vi "UTC KML time.vi"() -> (14 "String":string)   [LabVIEW 2015, in "Biblioteka moduł map v3.lvlib" / "KML.lvlib"]
uses:
  KML.lvlib
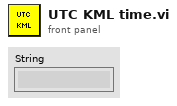
[diagram p1: front panel]
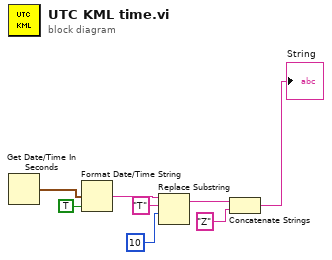
[diagram p0: block diagram]
diagram:
  n1 = Get Date/Time In Seconds() -> (seconds since 1Jan1904=w1:timestamp)
  n2 = Format Date/Time String(seconds (now)=w1, UTC format=TRUE) -> (date/time string=w2:string)  [unwired: 1 in]
  n3 = Replace Substring(3:10 ("offset (0)"), 4:"T" ("substring (\"\")"), 5:w2) -> (1:w7:string)  [unwired: 1 in, 1 out]
  n4 = Concatenate Strings(w7, "Z" ("string")) -> (→"String":string)
